vi "Do Request.vi"(7 "Processing In":refnum<class "Processing.lvclass">, 11 "Test WebSocket Page Controller in":refnum<class "Test WebSocket Page Controller.lvclass">) -> (0 "error out":errorcluster, 5 "Processing":refnum<class "Processing.lvclass">)   [LabVIEW 2020, in "Test WebSocket Page Controller.lvclass"]
uses:
  Test WebSocket Page Controller.lvclass
  Test WebSocket Page Controller.lvclass/Test WebSocket Page Controller.ctl
  <vilib>/IlluminatedG/IG HTTP Utils/HTTP Utils/Response/Response.lvclass
  HTTP Server/Processing/Processing.lvclass
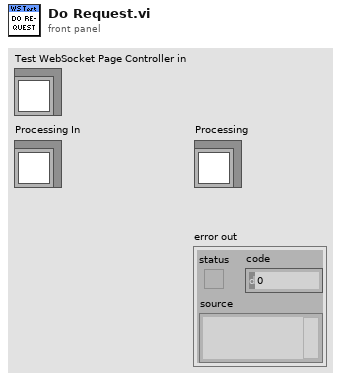
[diagram p1: front panel]
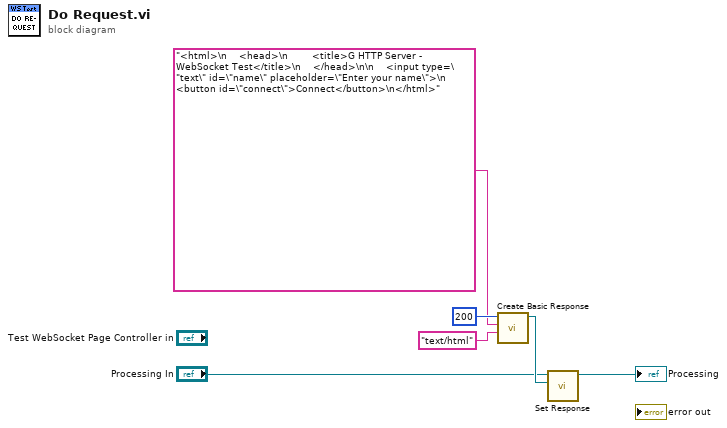
[diagram p0: block diagram]
diagram:
  n1 = call <vilib>:"Create Basic Response.vi"("Content-Type (text/plain)"="text/html", "Payload"="<html>\n    <head>\n        <title>G HTTP Server - WebSocket Test</title>\n    </head>\n\n    <input type=\"text\" id=\"name\" placeholder=\"Enter your name\">\n    <button id=\"connect\">Connect</button>\n</html>", "Status Code"=u16 200) -> ("Response out"=w3:refnum<class "Response.lvclass">)  [unwired: 7 in, 1 out]
  n2 = call "Set Response.vi"("Response"=w3, "Processing in"="Processing In") -> ("Processing out"=→"Processing":refnum<class "Processing.lvclass">)  [unwired: 9 in]
